vi "GetOutputPath.vi"(11 "Path":path) -> (3 "Output Path":path)   [LabVIEW 2017]
uses:
  FilesAndOutputPathMap.vi
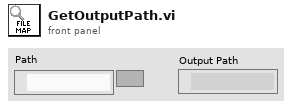
[diagram p1: front panel]
types:
  T1 = typedef "SourceJsonPaths.ctl" = cluster{"File to convert":path, "Output directory":path}
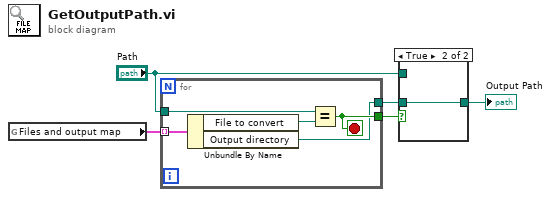
[diagram p0: block diagram]
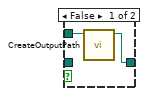
[diagram p2: hidden frame]
diagram:
  n1 = global read "FilesAndOutputPathMap.vi" "Files and output map"() -> (w5:T1[])
  n2 = for {
    tunnel: w5 -> [w9] mode=indexing
    tunnel: "Path" -> [w10]
    tunnel: [w8] -> w4
    tunnel: [w6] -> w1
    stop <- w8 stop-if-true
    n3 = Unbundle By Name(w9) -> ("File to convert"=w7:path, "Output directory"=w6:path)
    n4 = Equal?(x=w10, y=w7) -> (x = y?=w8:bool)
  }
  n5 = case shown="True" w4 {
    tunnel: "Path" -> [w12 _]
    tunnel: [w11 w13] -> w3
    tunnel: w1 -> [_ w13]
    frame False {
      n6 = call "CreateOutputPath.vi"("File to convert"=w12) -> ("appended path"=w11:path)  [unwired: 9 in, 1 out]
    }
    frame True {
    }
  }
  "Output Path" <- w3
